vi "testing_sleep_sweep.vi"() -> ()   [LabVIEW 2015, in "Tausand AB1000.lvlib"]
uses:
  <instrlib>/Tausand AB1000/Tausand AB1000.lvlib
  <instrlib>/Tausand AB1000/Public/Controls/deviceTypeRing.ctl
  <instrlib>/Tausand AB1000/Public/Controls/channelRing.ctl
  <instrlib>/Tausand AB1000/Public/Controls/counters4ch.ctl
panel:
  in  "sleep step":i32(ring)=1 items=["1ns"=1, "2ns"=2, "5ns"=5, "10ns"=10]
  out "counts Chart":T1(graph)
  out "Final data":u32[][](array[numeric])
  in  "max sleep":i32=100
  out "sleep Chart":u32(graph)
  in  "stop":bool
  out "this i":i32
  in  "data per sleep":i32=10
  in  "VISA resource name":refnum<visa-resource-name>
  out "current data":T2
  in  "sampling (ms)":u32=1000
  in  "channel to sweep":T3=1 items=["none", "A", "B", "C", "D", "E", "F", "G", "H"]
  out "this sleep":i32
  in  "device type":T4 items=["any"=0, "AB1002"=1002, "AB1004"=1004, "AB1502"=1502, "AB1504"=1504, "AB1902"=1902, "AB1904"=1904]
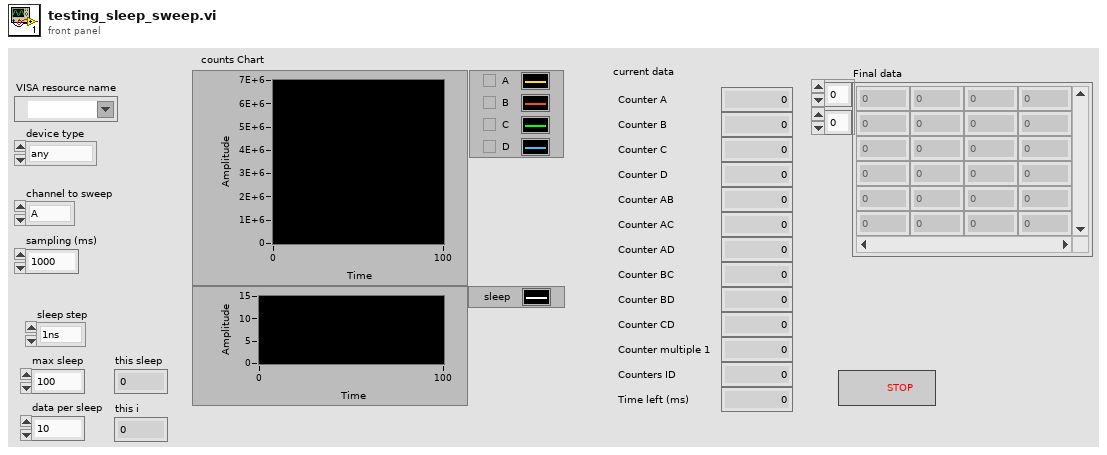
[diagram p1: front panel]
types:
  T1 = cluster{"counter_A":u32, "counter_B":u32, "counter_C":u32, "counter_D":u32, "counter_AB":u32, "counter_AC":u32, "counter_AD":u32, "counter_BC":u32, "counter_BD":u32, "counter_CD":u32, "counter_multiple_1":u32, "counters_ID":u32, "time_left":u32}
  T2 = typedef "Tausand AB1000.lvlib/counters4ch.ctl" = cluster{"counter_A":u32, "counter_B":u32, "counter_C":u32, "counter_D":u32, "counter_AB":u32, "counter_AC":u32, "counter_AD":u32, "counter_BC":u32, "counter_BD":u32, "counter_CD":u32, "counter_multiple_1":u32, "counters_ID":u32, "time_left":u32}
  T3 = typedef "Tausand AB1000.lvlib/channelRing.ctl" = u8
  T4 = typedef "Tausand AB1000.lvlib/deviceTypeRing.ctl" = u16
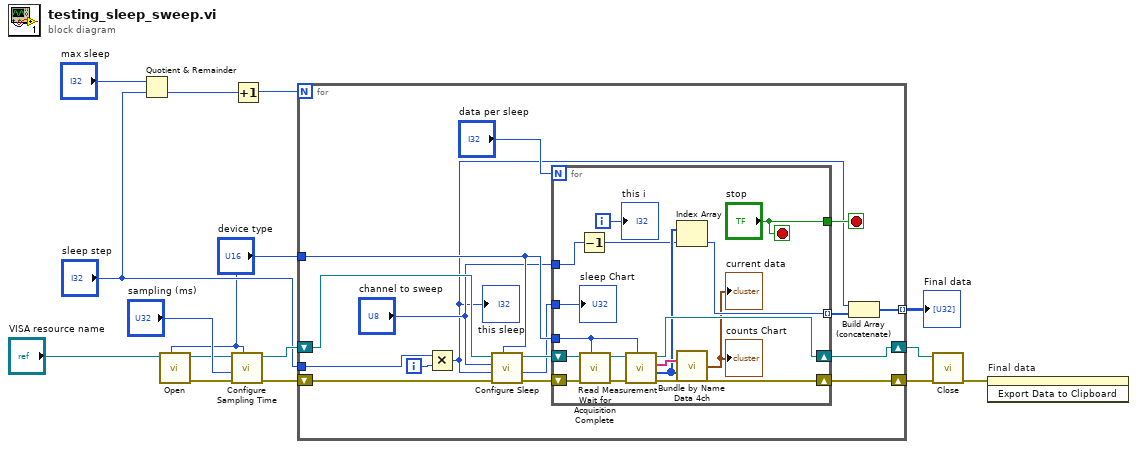
[diagram p0: block diagram]
diagram:
  n1 = Quotient & Remainder(x="max sleep", y="sleep step") -> (floor(x/y)=w2:i32)  [unwired: 1 out]
  n2 = call <instrlib>:"Open.vi"("device type (any)"="device type", "VISA resource name"="VISA resource name") -> ("error out"=w10:errorcluster, "VISA resource name out"=w12:refnum<visa-resource-name>)  [unwired: 8 in]
  n3 = call <instrlib>:"Configure Sampling Time.vi"("device type"="device type", "error in (no error)"=w10, "value (1000 ms)"="sampling (ms)", "VISA Refnum in"=w12) -> ("error out"=w9:errorcluster, "VISA Refnum out"=w11:refnum<visa-resource-name>)  [unwired: 5 in, 1 out]
  n4 = Increment(x=w2) -> (x+1=w6:i32)
  n5 = for {
    N: w6 -> [_]
    tunnel: "device type" -> [w29]
    shift-right: [w26] -> w14
    shift-left: w11 -> [w31]
    shift-right: [w25] -> w15
    shift-left: w9 -> [w30]
    tunnel: [w19] -> w7 mode=indexing
    tunnel: "sleep step" -> [w16]
    i -> [w18]
    stop <- w23 stop-if-true
    n6 = Multiply(x=w16, y=w18) -> (x*y=w17:i32)
    "this sleep" <- w17
    n7 = call <instrlib>:"Configure Sleep.vi"("device type"=w29, "error in (no error)"=w30, "value (0 ns)"=w17, "channel"="channel to sweep", "VISA Refnum in"=w31) -> ("error out"=w27:errorcluster, "value ns out"=w22:u32, "VISA Refnum out"=w28:refnum<visa-resource-name>)  [unwired: 4 in]
    n8 = for {
      N: "data per sleep" -> [_]
      tunnel: w29 -> [w32]
      shift-right: [w43] -> w26
      shift-left: w28 -> [w47]
      shift-right: [w42] -> w25
      shift-left: w27 -> [w46]
      tunnel: ["stop"] -> w23
      tunnel: w22 -> [w38]
      tunnel: "channel to sweep" -> [w35]
      tunnel: [w34] -> w20 mode=indexing
      i -> [w40]
      stop <- "stop" stop-if-true
      n9 = Decrement(x=w35) -> (x-1=w36:T3)
      n10 = call <instrlib>:"Wait for Acquisition Complete.vi"("device type"=w32, "error in (no error)"=w46, "VISA resource name"=w47) -> ("error out"=w45:errorcluster, "VISA resource name out"=w44:refnum<visa-resource-name>)  [unwired: 7 in]
      n11 = call <instrlib>:"Read Measurement.vi"("device type"=w32, "error in (no error)"=w45, "VISA Refnum in"=w44) -> ("error out"=w42:errorcluster, "values"=w37:u32[], "labels"=w41:string[], "VISA Refnum out"=w43:refnum<visa-resource-name>)  [unwired: 3 in, 2 out]
      n12 = Index Array(array=w37, index=w36) -> (element=w34:u32)
      n13 = call <instrlib>:"Bundle by Name Data 4ch.vi"("names"=w41, "values"=w37) -> ("output cluster 4ch"=→"current data" →"counts Chart":T2)  [unwired: 13 in]
      "this i" <- w40
      "sleep Chart" <- w38
    }
    n14 = Build Array (concatenate)(w17, w20) -> (w19:u32[])
  }
  "Final data" <- w7
  n15 = call <instrlib>:"Close.vi"("error in (no error)"=w15, "VISA resource name"=w14) -> ("error out"=w5:errorcluster)  [unwired: 9 in]
  n16 = invoke on="Final data" class="Arr (strict)" method="Export Data to Clipboard"(error in=w5) -> ()  [unwired: 2 in, 3 out]
